vi "Read Device Config.vi"(8 "error in (no error)":errorcluster, 11 "Configuration in":refnum<class "Configuration.lvclass">) -> (0 "error out":errorcluster, 1 "Values":string[](array[string]), 2 "Keys":string[](array[string]), 3 "Configuration out":refnum<class "Configuration.lvclass">)   [LabVIEW 2023, in "Configuration.lvlib" / "Configuration.lvclass"]
uses:
  Library/Configuration.lvclass
  Library/Configuration.lvclass/Configuration.ctl
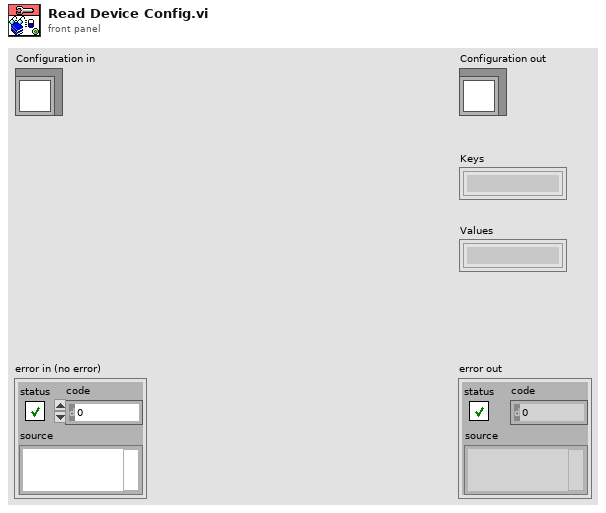
[diagram p1: front panel]
types:
  T1 = typedef "Configuration.lvlib/Configuration.lvclass/Definitions.ctl" = map{string, T2}
  T2 = typedef "Configuration.lvlib/Configuration.lvclass/Config.ctl" = map{string, string}
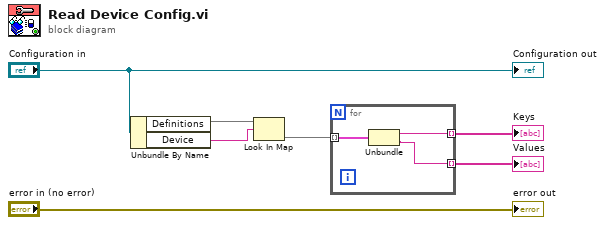
[diagram p0: block diagram]
diagram:
  n1 = Unbundle By Name("Configuration in") -> ("Definitions"=w5:T1, "Device"=w4:string)
  n2 = Look In Map(map=w5, key=w4) -> (value=w3:T2)  [unwired: 1 in, 1 out]
  n3 = for {
    tunnel: w3 -> [w10] mode=indexing
    tunnel: [w9] -> w2 mode=indexing
    tunnel: [w8] -> w1 mode=indexing
    n4 = Unbundle(w10) -> ("Key"=w9:string, "Value"=w8:string)
  }
  "Keys" <- w2
  "Values" <- w1
  "error out" <- "error in (no error)"
  "Configuration out" <- "Configuration in"
